vi "DisableCell.vi"(0 "Column in":refnum<class "Column.lvclass">, 5 "Cell Position":T1, 7 "Table Data in":string[][](array[string]), 9 "Table CtlRef In":refnum<vi>, 11 "error in (no error)":errorcluster) -> (4 "Column out":refnum<class "Column.lvclass">, 8 "Table Data out":string[][](array[string]), 10 "Table CtlRef Out":refnum<vi>, 15 "error out":errorcluster)   [LabVIEW 2013, in "Column.lvclass"]
uses:
  Column.lvclass
  <vilib>/Utility/miscctls.llb/LVRowAndColumnTypeDef.ctl
  Column.lvclass/Column.ctl
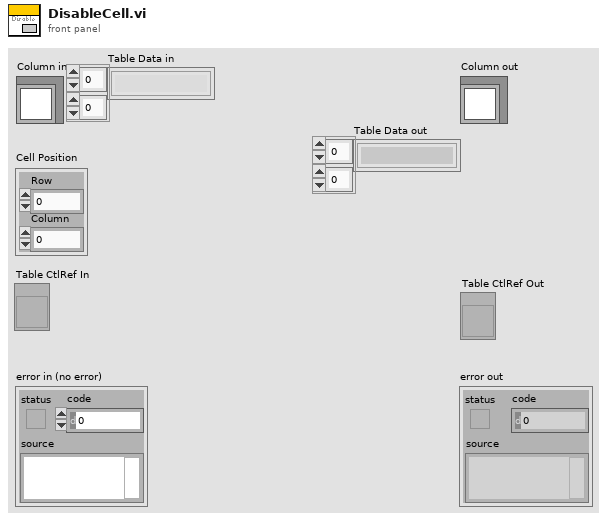
[diagram p1: front panel]
types:
  T1 = typedef "LVRowAndColumnTypeDef.ctl" = cluster{"Row":i32, "Column":i32}
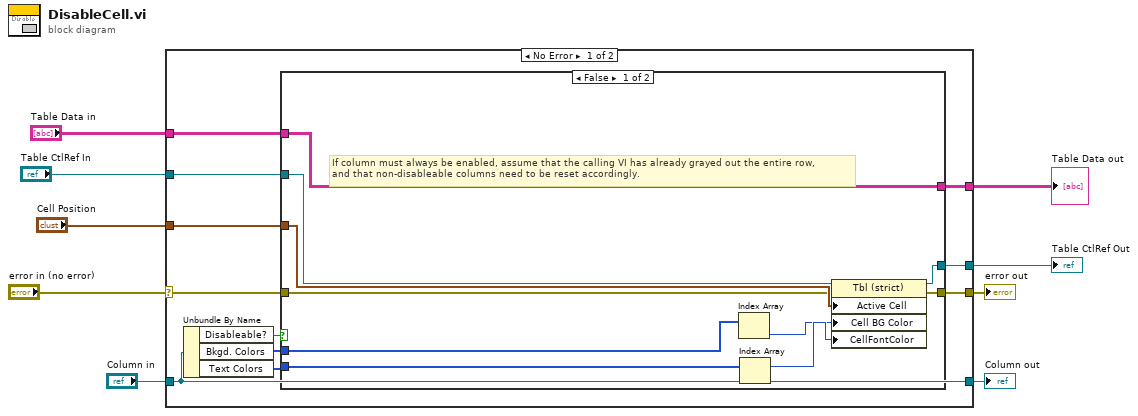
[diagram p0: block diagram]
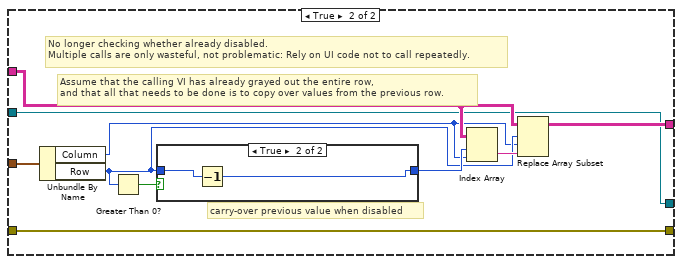
[diagram p2: hidden frame]
diagram:
  n1 = case shown="No Error" "error in (no error)" {
    selector: "error in (no error)" -> [w17 w47]
    tunnel: [w16 w47] -> w8
    tunnel: [w15 w46] -> w6
    tunnel: "Column in" -> [w15 w46]
    tunnel: "Cell Position" -> [w18 _]
    tunnel: "Table CtlRef In" -> [w20 w45]
    tunnel: [w19 w45] -> w3
    tunnel: "Table Data in" -> [w13 w44]
    tunnel: [w12 w44] -> w1
    frame No Error {
      n2 = Unbundle By Name(w15) -> ("Disableable?"=w14:bool, "Bkgd. Colors"=w11:u32[], "Text Colors"=w10:u32[])
      n3 = case shown="False" w14 {
        tunnel: w20 -> [w29 w31]
        tunnel: [w28 w31] -> w19
        tunnel: w18 -> [w27 w40]
        tunnel: w17 -> [w26 w32]
        tunnel: [w25 w32] -> w16
        tunnel: w13 -> [w30 w37]
        tunnel: [w30 w33] -> w12
        tunnel: w11 -> [w24 _]
        tunnel: w10 -> [w23 _]
        frame False {
          # "If column must always be enabled, assume that the calling VI has already grayed out the entire row,\nand that non-disableable columns need to be reset accordingly."
          n4 = Index Array(array=w24) -> (element=w21:u32)  [unwired: 1 in]
          n5 = Index Array(array=w23) -> (element=w22:u32)  [unwired: 1 in]
          n6 = property class="Tbl (strict)"(reference=w29, error in=w26, "Active Cell"=w27, "Cell BG Color"=w21, "CellFontColor"=w22) -> (reference out=w28:refnum<vi>, error out=w25:errorcluster)
        }
        frame True {
          # "Assume that the calling VI has already grayed out the entire row,\nand that all that needs to be done is to copy over values from the previous row."
          # "No longer checking whether already disabled. \nMultiple calls are only wasteful, not problematic: Rely on UI code not to call repeatedly."
          # "carry-over previous value when disabled"
          n7 = Unbundle By Name(w40) -> ("Column"=w34:i32, "Row"=w35:i32)
          n8 = Greater Than 0?(x=w35) -> (x > 0?=w38:bool)
          n9 = case shown="True" w38 {
            tunnel: [w41 w43] -> w39
            tunnel: w35 -> [w41 w42]
            frame False {
            }
            frame True {
              n10 = Decrement(x=w42) -> (x-1=w43:i32)
            }
          }
          n11 = Index Array(array=w37, index (row)=w39, index (col)=w34) -> (element=w36:string)
          n12 = Replace Array Subset(array=w37, new element=w36, index (row)=w35, index (col)=w34) -> (w33:string[][])
        }
      }
    }
    frame Error {
    }
  }
  "error out" <- w8
  "Column out" <- w6
  "Table CtlRef Out" <- w3
  "Table Data out" <- w1
